vi "SVT Weighting Filter (octave) (N Ch).vi"(0 "octave spectra":T5(array[cluster]) {"band power" format="%.2f"; "nominal frequencies [Hz]" format="%.2f"}, 5 "weighting":u16(ring) items=["Linear", "A-weighting", "B-weighting", "C-weighting"], 9 "octave info in":T1[](array[typedef]) {"engineering units" items=["custom..."=0, "V"=1, "A"=21, "C"=30, "pC"=31, "s"=32, "-"=29, "Pa"=2, "N"=20, "g"=3, "m/s^2"=4, "m/s"=5, "m"=6, "mm/s"=12, "mm"=13, "micron/s"=14, "micron"=15, "in/s^2"=7, "in/s"=8, "in"=9, "mil/s"=10, "mil"=11, "rad/s^2"=16, "rad/s"=17, "rad"=18, "deg/s^2"=26, "deg/s"=27, "deg"=28, "RPM"=22, "cycle/s^2"=23, "Hz"=24, "cycle"=25, "strain"=19]; "dB reference" format="%.2e"; "weighting filter" items=["Linear", "A-weighting", "B-weighting", "C-weighting", "ITU-R 468-4", "Dolby", "CCITT", "C-message", "Wb", "Wc", "Wd", "We", "Wf", "Wh", "Wj", "Wk", "Wm", "AES17 20 kHz lowpass", "AES17 40 kHz lowpass", "AES17 20 kHz highpass", "AES17 40 kHz highpass"]}, 11 "error in (no error)":errorcluster) -> (4 "weighted octave spectra":T5(array[cluster]) {"band power" format="%.2f"; "nominal frequencies [Hz]" format="%.2f"}, 6 "unit labels":string[](array[string]), 8 "total band powers":dbl[](array[numeric]) format="%.2f", 10 "octave info out":T1[](array[typedef]) {"engineering units" items=["custom..."=0, "V"=1, "A"=21, "C"=30, "pC"=31, "s"=32, "-"=29, "Pa"=2, "N"=20, "g"=3, "m/s^2"=4, "m/s"=5, "m"=6, "mm/s"=12, "mm"=13, "micron/s"=14, "micron"=15, "in/s^2"=7, "in/s"=8, "in"=9, "mil/s"=10, "mil"=11, "rad/s^2"=16, "rad/s"=17, "rad"=18, "deg/s^2"=26, "deg/s"=27, "deg"=28, "RPM"=22, "cycle/s^2"=23, "Hz"=24, "cycle"=25, "strain"=19]; "dB reference" format="%.2e"; "weighting filter" items=["Linear", "A-weighting", "B-weighting", "C-weighting", "ITU-R 468-4", "Dolby", "CCITT", "C-message", "Wb", "Wc", "Wd", "We", "Wf", "Wh", "Wj", "Wk", "Wm", "AES17 20 kHz lowpass", "AES17 40 kHz lowpass", "AES17 20 kHz highpass", "AES17 40 kHz highpass"]}, 15 "error out":errorcluster)   [LabVIEW 2017, in "SoundVib_ABCWeighting.lvlib"]
doc: "Applies the selected weighting to a previously computed <B>octave spectrum</B> or <B>octave spectra</B>. This VI weights each spectral bin according to the attenuation of the specified filter at the bin center frequency. You can use this VI in a loop to process multiple blocks. Wire data to the <B>octave spectrum</B> input to determine the polymorphic instance to use or manually select the instance."
uses:
  <vilib>/addons/Sound and Vibration/svt_Weighting/SoundVib_ABCWeighting.lvlib
  <vilib>/addons/_NISVFA/_Shared subVIs/Controls/svc_Octave Info.ctl
  <vilib>/addons/_NISVFA/_Shared subVIs/Controls/svc_Octave Standard.ctl
  <vilib>/addons/_NISVFA/_Shared subVIs/Controls/svc_Weighting Filter Text Ring.ctl
  <vilib>/addons/_NISVFA/_Shared subVIs/Controls/svc_Engineering Units Text Ring.ctl
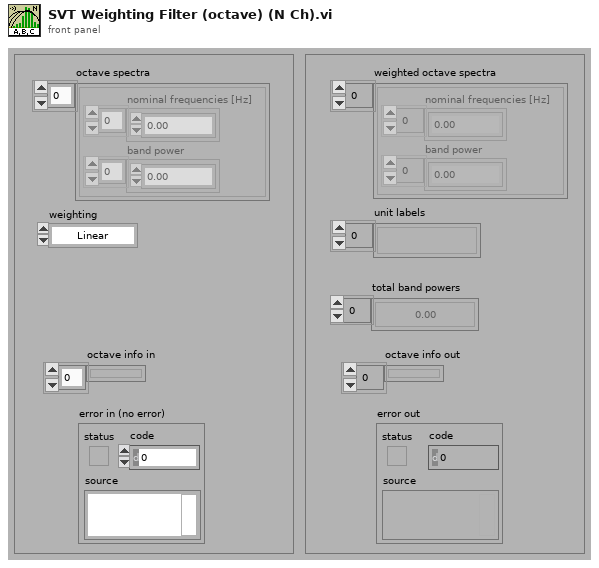
[diagram p1: front panel]
types:
  T1 = typedef "svc_Octave Info.ctl" = cluster{"standard":T2, "bandwidth":enum16{"1 octave", "1/3 octave", "1/6 octave", "1/12 octave", "1/24 octave"}, "low band":i32, "high band":i32, "weighting filter":T3, "dB reference":dbl, "dB On":bool, "unit label":string, "channel name":string, "description":string, "engineering units":T4, "custom label":string, "spectrum type":enum16{"power", "magnitude"}, "spectral density":bool, "filters settled":bool}
  T2 = typedef "svc_Octave Standard.ctl" = enum16{"ANSI S1.11", "IEC 61260"}
  T3 = typedef "svc_Weighting Filter Text Ring.ctl" = u16
  T4 = typedef "svc_Engineering Units Text Ring.ctl" = u16
  T5 = cluster{"nominal frequencies [Hz]":dbl[], "band power":dbl[]}[]
  T6 = cluster{"nominal frequencies [Hz]":dbl[], "band power":dbl[]}
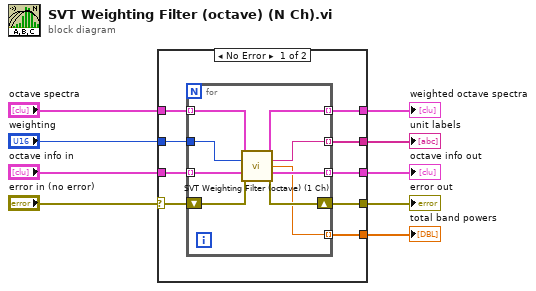
[diagram p0: block diagram]
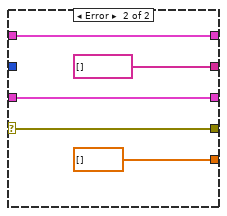
[diagram p2: hidden frame]
diagram:
  n1 = case shown="No Error" "error in (no error)" {
    selector: "error in (no error)" -> [w17 w32]
    tunnel: [w14 w32] -> w8
    tunnel: "weighting" -> [w18 _]
    tunnel: [w12 string[] []] -> w6
    tunnel: "octave spectra" -> [w16 w30]
    tunnel: [w13 w30] -> w4
    tunnel: "octave info in" -> [w15 w29]
    tunnel: [w11 w29] -> w2
    tunnel: [w10 dbl[] []] -> w1
    frame No Error {
      n2 = for {
        tunnel: w18 -> [w27]
        tunnel: w16 -> [w26] mode=indexing
        tunnel: w15 -> [w25] mode=indexing
        tunnel: [w22] -> w13 mode=indexing
        tunnel: [w21] -> w12 mode=indexing
        tunnel: [w20] -> w11 mode=indexing
        shift-right: [w23] -> w14
        shift-left: w17 -> [w24]
        tunnel: [w19] -> w10 mode=indexing
        n3 = call <vilib>:"SVT Weighting Filter (octave) (1 Ch).vi"("octave spectrum"=w26, "weighting"=w27, "octave info in"=w25, "error in (no error)"=w24) -> ("weighted octave spectrum"=w22:T6, "unit label"=w21:string, "total band power"=w19:dbl, "octave info out"=w20:T1, "error out"=w23:errorcluster)  [unwired: 7 in]
      }
    }
    frame Error {
      (unwired) "" ("Unit label (in)")
    }
  }
  "error out" <- w8
  "unit labels" <- w6
  "weighted octave spectra" <- w4
  "octave info out" <- w2
  "total band powers" <- w1
